vi "Autonomous Independent.vi"() -> ()   [LabVIEW 2015]
doc: "This VI is called when autonomous begins, and will automatically be terminated when autonomous ends. You can carry out timed or sensor driven robot movement independently without needing to return to the caller."
uses:
  <vilib>/Rock Robotics/WPI/Utilities/WPI_GetSetVariantRefNum.vi
  <vilib>/Rock Robotics/Network Tables/NT Write Numeric Array.vi
  <vilib>/Rock Robotics/Network Tables/NT Read String.vi
  Robot Motor Controllers.llb/RobotGlobalVariables.vi
  <vilib>/Rock Robotics/WPI/RobotDrive/WPI_RobotDriveArcadeDrive_Standard(NoSaturation).vi
  <vilib>/Rock Robotics/Network Tables/NT Write Boolean.vi
panel:
  out "Current Movement, for debugging 2":T1 {"Y Joystick Value" scale=1.0..-1.0; "X Joystick Value" scale=-1.0..1.0}
  in  "Array of robot movements 2":T2(array[cluster])=[{"X Joystick Value"=0.39393939393939403, "Y Joystick Value"=0.0, "Delay (sec)"=1.0, "Movement Name"="turn"}, {"X Joystick Value"=-0.3737373737373737, "Y Joystick Value"=0.0, "Delay (sec)"=1.0, "Movement Name"="turn back"}] {"Y Joystick Value" scale=1.0..-1.0; "X Joystick Value" scale=-1.0..1.0}
  out "Current Movement, for debugging":T1 {"Y Joystick Value" scale=1.0..-1.0; "X Joystick Value" scale=-1.0..1.0}
  in  "Array of robot movements":T2(array[cluster])=[{"X Joystick Value"=0.39393939393939403, "Y Joystick Value"=0.0, "Delay (sec)"=1.0, "Movement Name"="turn"}, {"X Joystick Value"=-0.3737373737373737, "Y Joystick Value"=0.0, "Delay (sec)"=1.0, "Movement Name"="turn back"}] {"Y Joystick Value" scale=1.0..-1.0; "X Joystick Value" scale=-1.0..1.0}
  # "Be sure to right-click and choose Data Operations>>Make Current Value default if you want to save the array values with the VI"
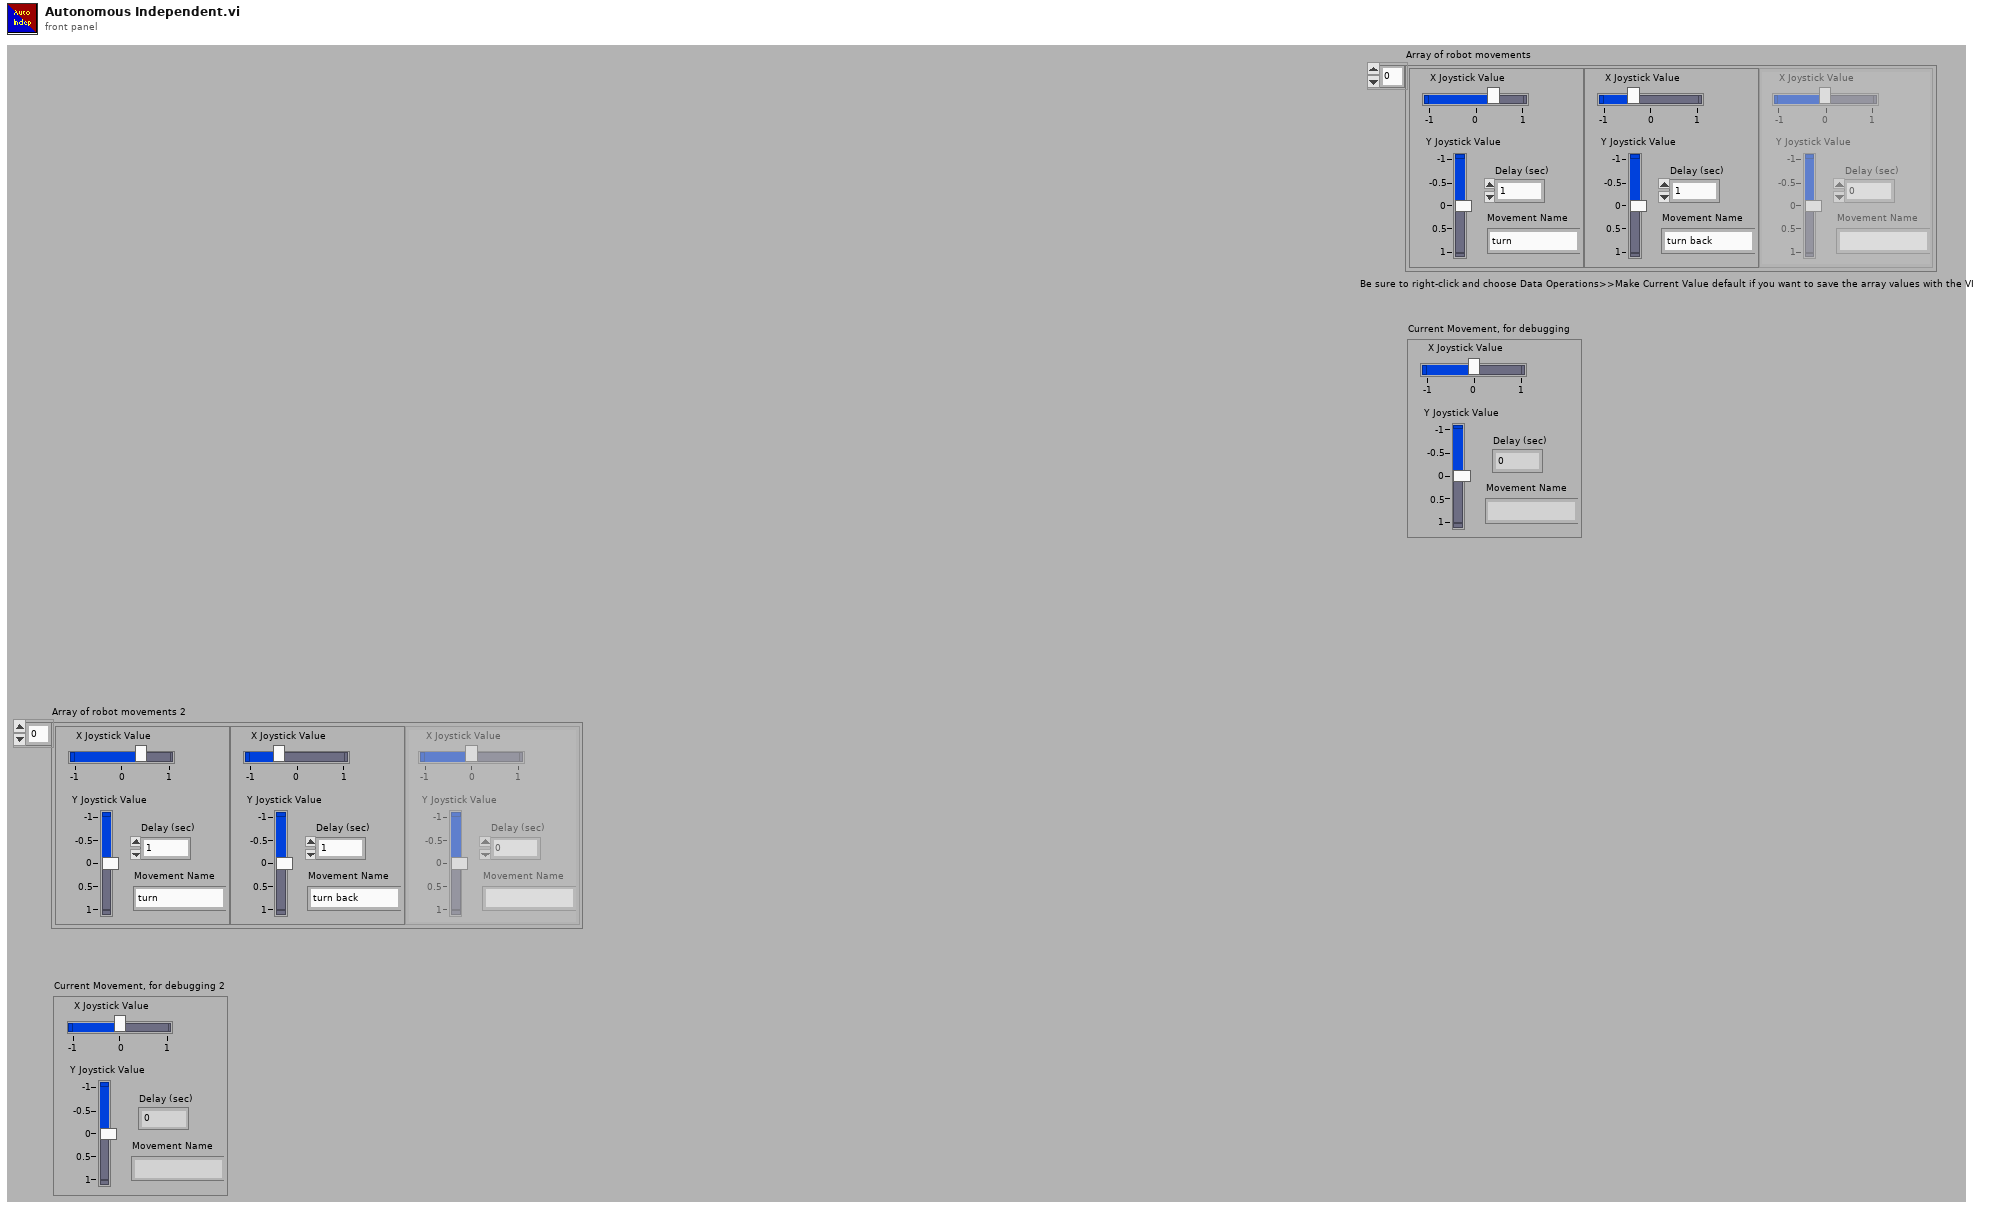
[diagram p1: front panel]
types:
  T1 = cluster{"X Joystick Value":dbl, "Y Joystick Value":dbl, "Delay (sec)":dbl, "Movement Name":string}
  T2 = cluster{"X Joystick Value":dbl, "Y Joystick Value":dbl, "Delay (sec)":dbl, "Movement Name":string}[]
  T3 = typedef "WPI_RobotDriveDevRef.ctl" = cluster{"DevStatus":errorcluster, "Motors[]":T4[], "Square Inputs":bool, "Max Output":dbl}
  T4 = typedef "WPI_MotorControlDeviceRef.ctl" = cluster{"DeviceStatus":errorcluster, "Type":T5, "PWM":cluster{"PWM Channel":T6, "DeadBand":T7}, "CAN":cluster{"Device Number":u8, "Control Mode":T8, "Semaphore":T9, "Max Vout":dbl, "TalonSRX Control Mode":T10}, "Invert":bool}
  T5 = typedef "WPI_MotorControlType.ctl" = enum16{"PWM", "CAN", "CANTalonSRX"}
  T6 = typedef "FPGA_DIOPWMChannel.ctl" = enum8{"PWM 0", "PWM 1", "PWM 2", "PWM 3", "PWM 4", "PWM 5", "PWM 6", "PWM 7", "PWM 8", "PWM 9", "PWM MXP 0", "PWM MXP 1", "PWM MXP 2", "PWM MXP 3", "PWM MXP 4", "PWM MXP 5", "PWM MXP 6", "PWM MXP 7", "PWM MXP 8", "PWM MXP 9", "Invalid"}
  T7 = typedef "WPI_PWMDeadband.ctl" = cluster{"Name":string, "maxPositivePwm":i32, "minPositivePwm":i32, "centerPwm":i32, "maxNegativePwm":i32, "minNegativePwm":i32, "angularRange":u16}
  T8 = typedef "WPI_CANJaguar_ControlMode.ctl" = enum8{"Percent VBus", "Current", "Speed", "Position", "Voltage"}
  T9 = typedef "Semaphore RefNum" = refnum<k1>
  T10 = typedef "WPI_CANTalonSRX_APIControlMode.ctl" = enum8{"Percent VBus", "Speed", "Position", "Slave", "Unchanged / Invalid", "Voltage Compensation", "Current", "Motion Profile"}
  T11 = typedef "WPI_JoystickDevRef.ctl" = cluster{"Device":T12}
  T12 = typedef "WPI_JoystickDeviceEnum.ctl" = enum16{"USB 0", "USB 1", "USB 2", "USB 3", "USB 4", "USB 5"}
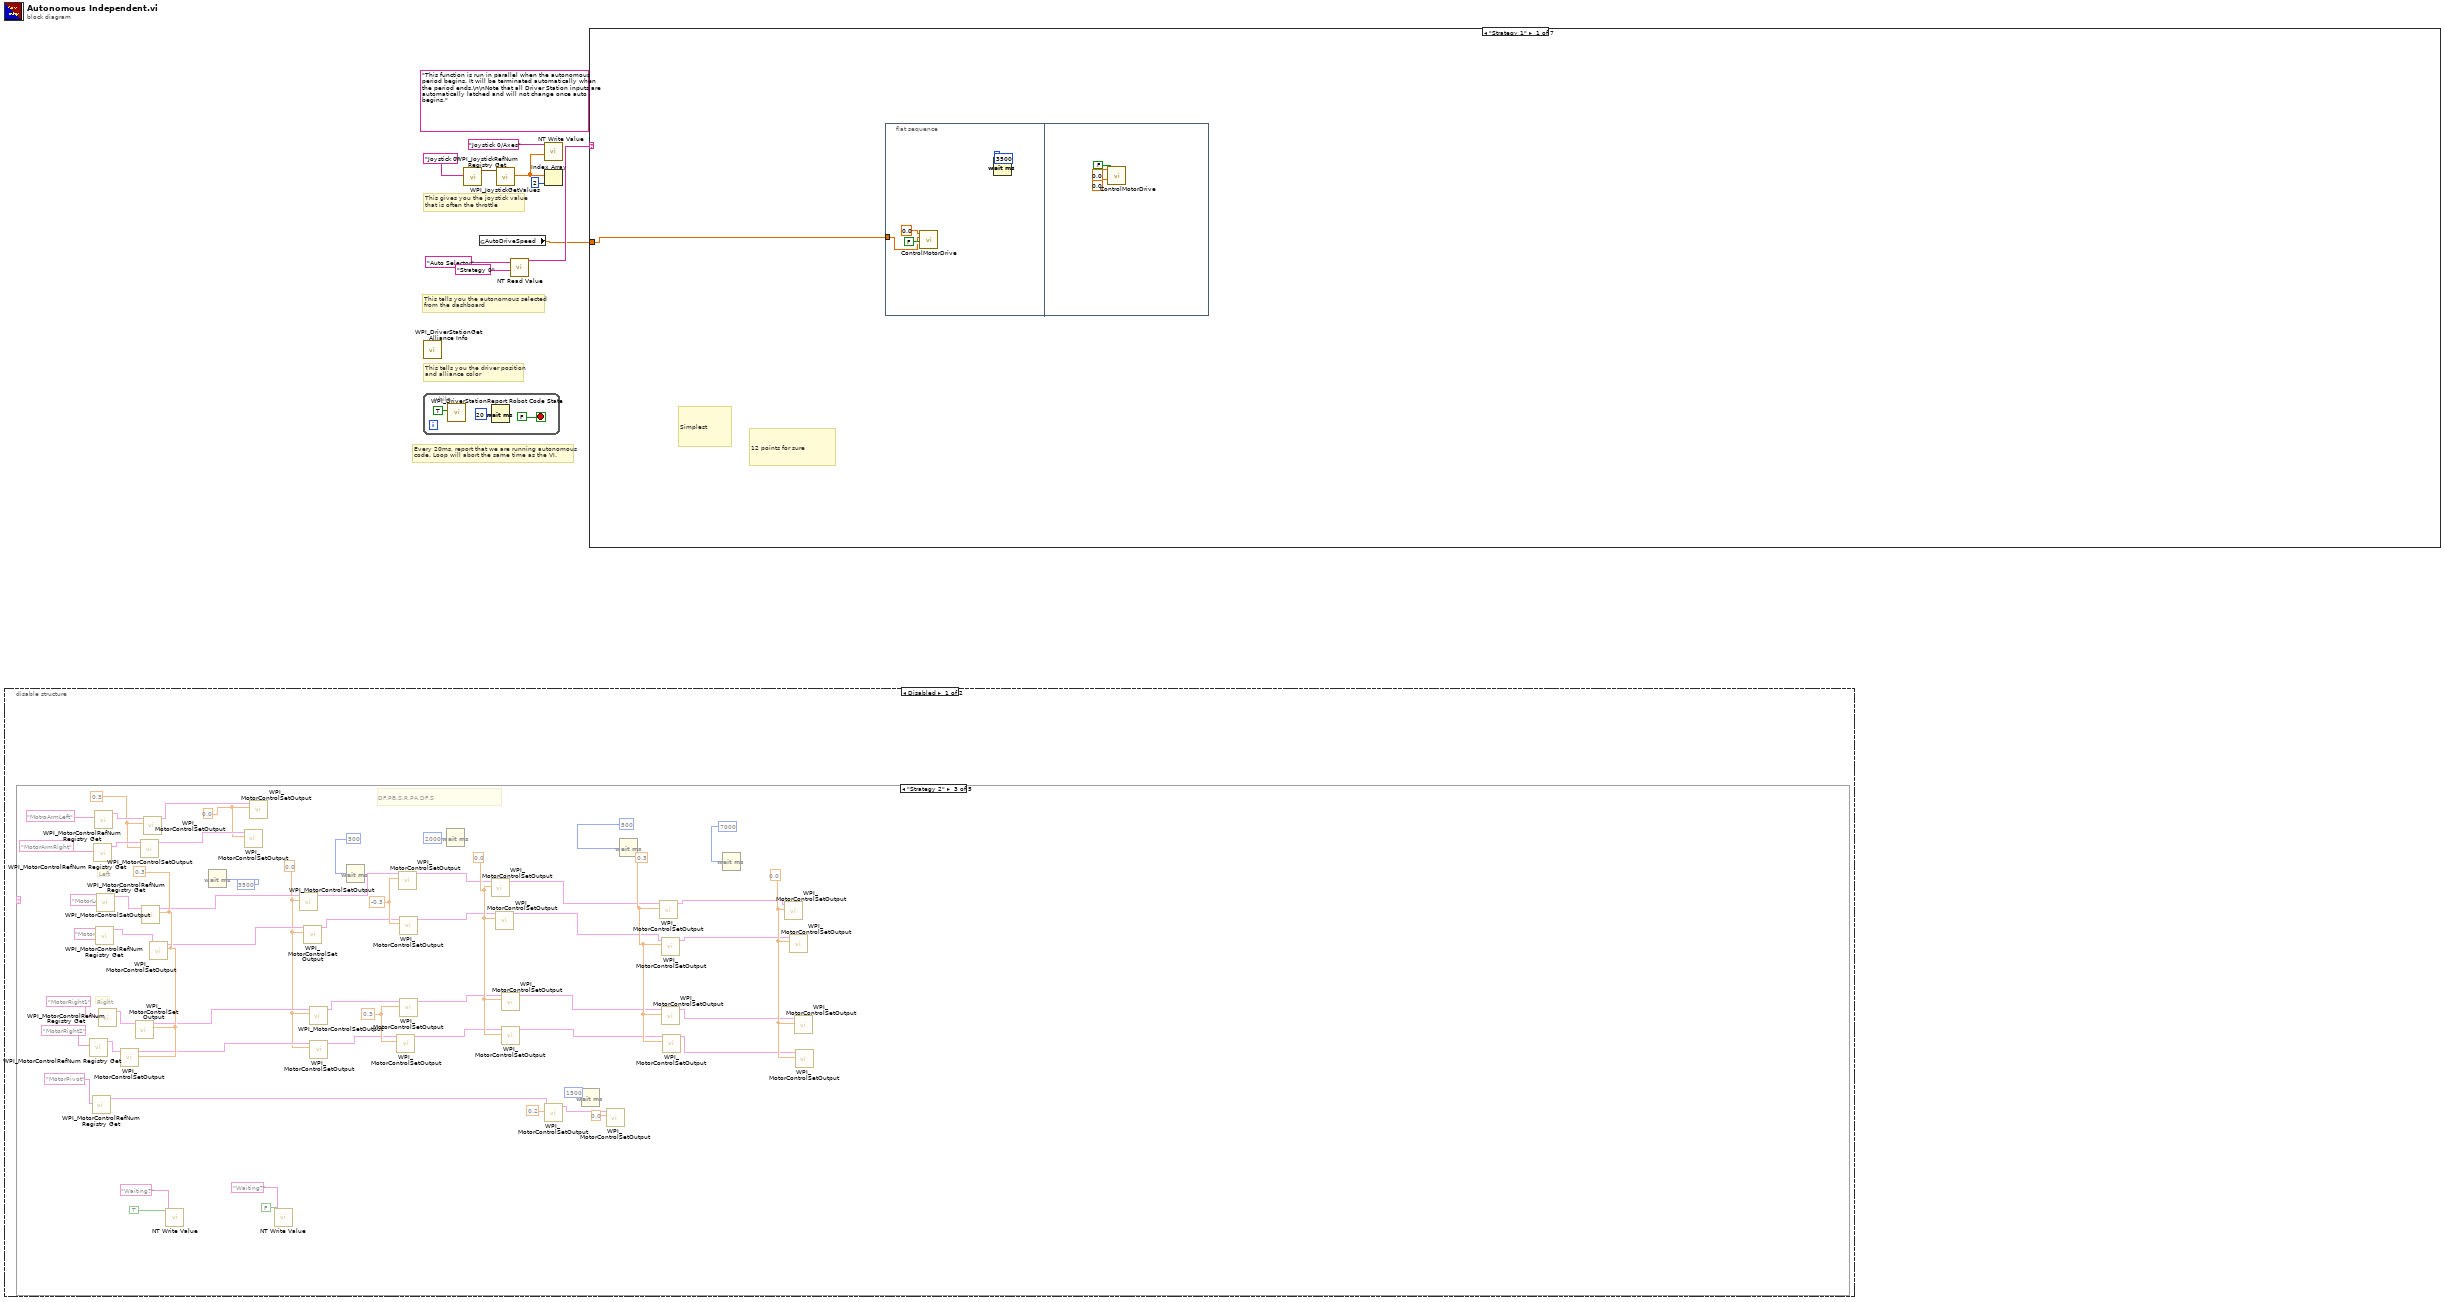
[diagram p0: block diagram]
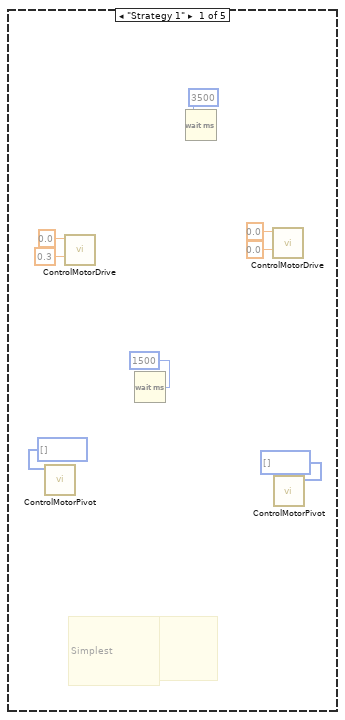
[diagram p2: hidden frame]
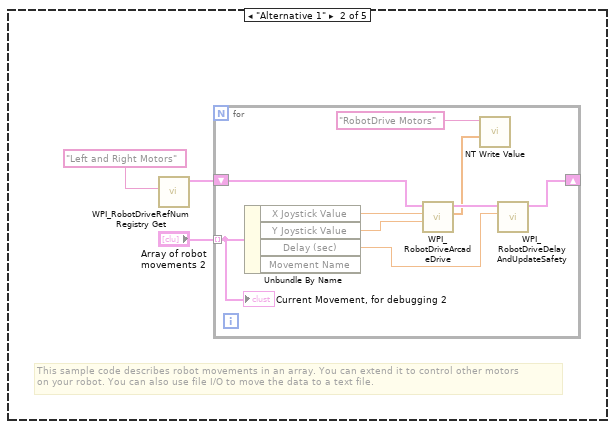
[diagram p3: hidden frame]
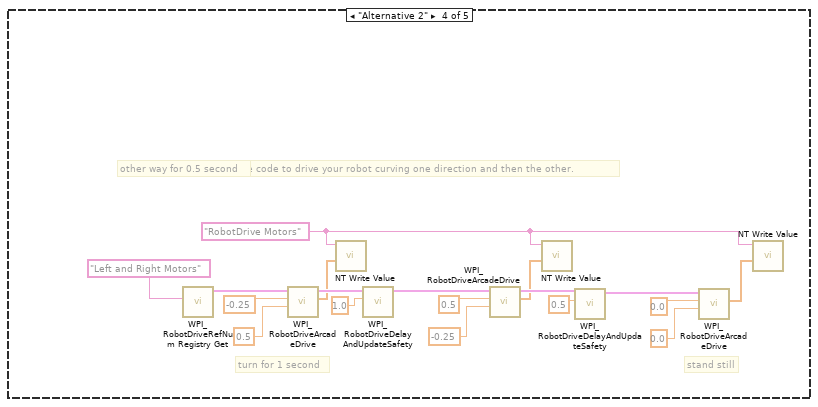
[diagram p4: hidden frame]
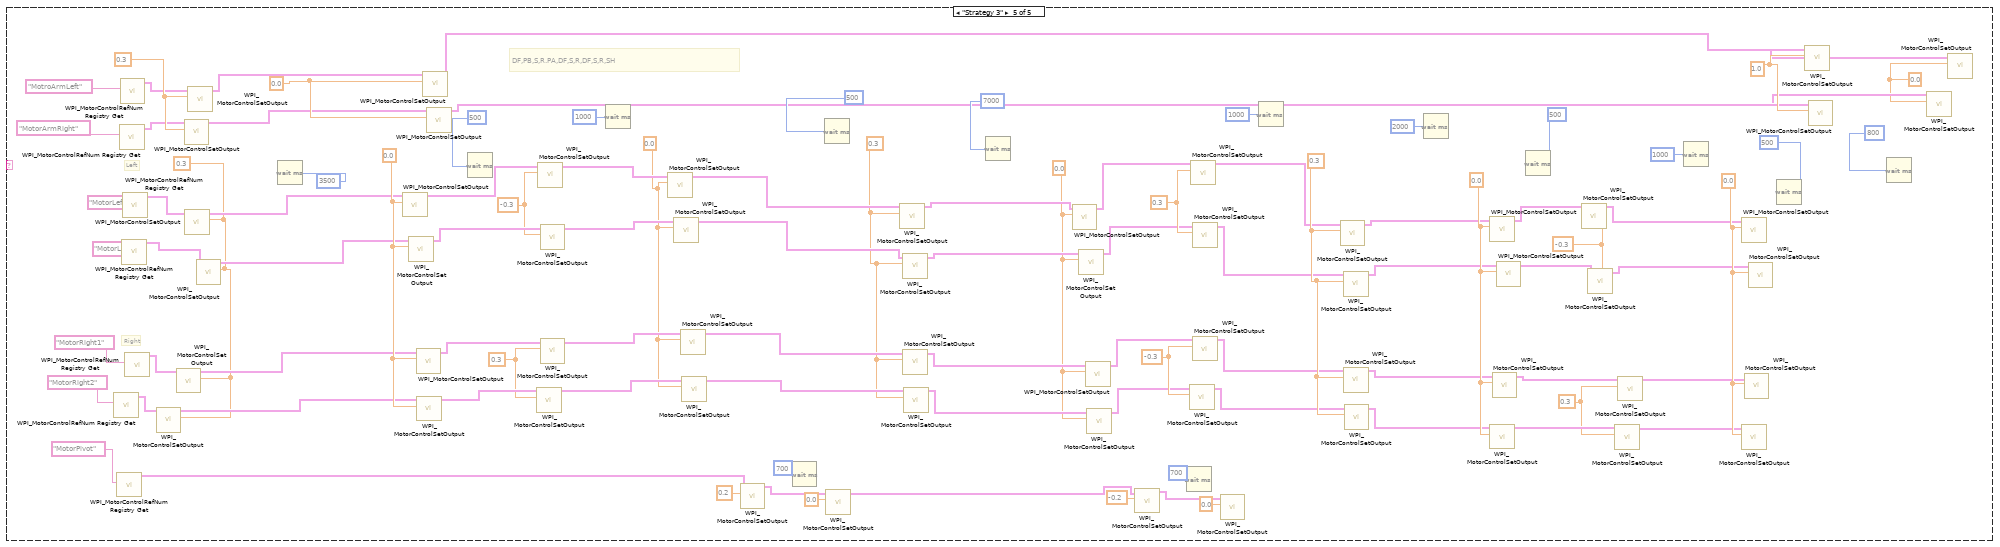
[diagram p5: hidden frame]
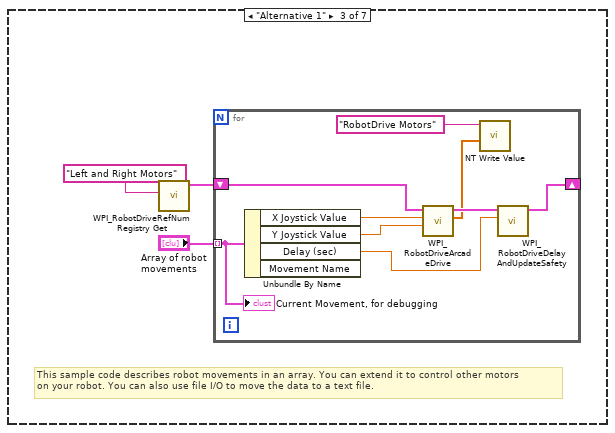
[diagram p8: hidden frame]
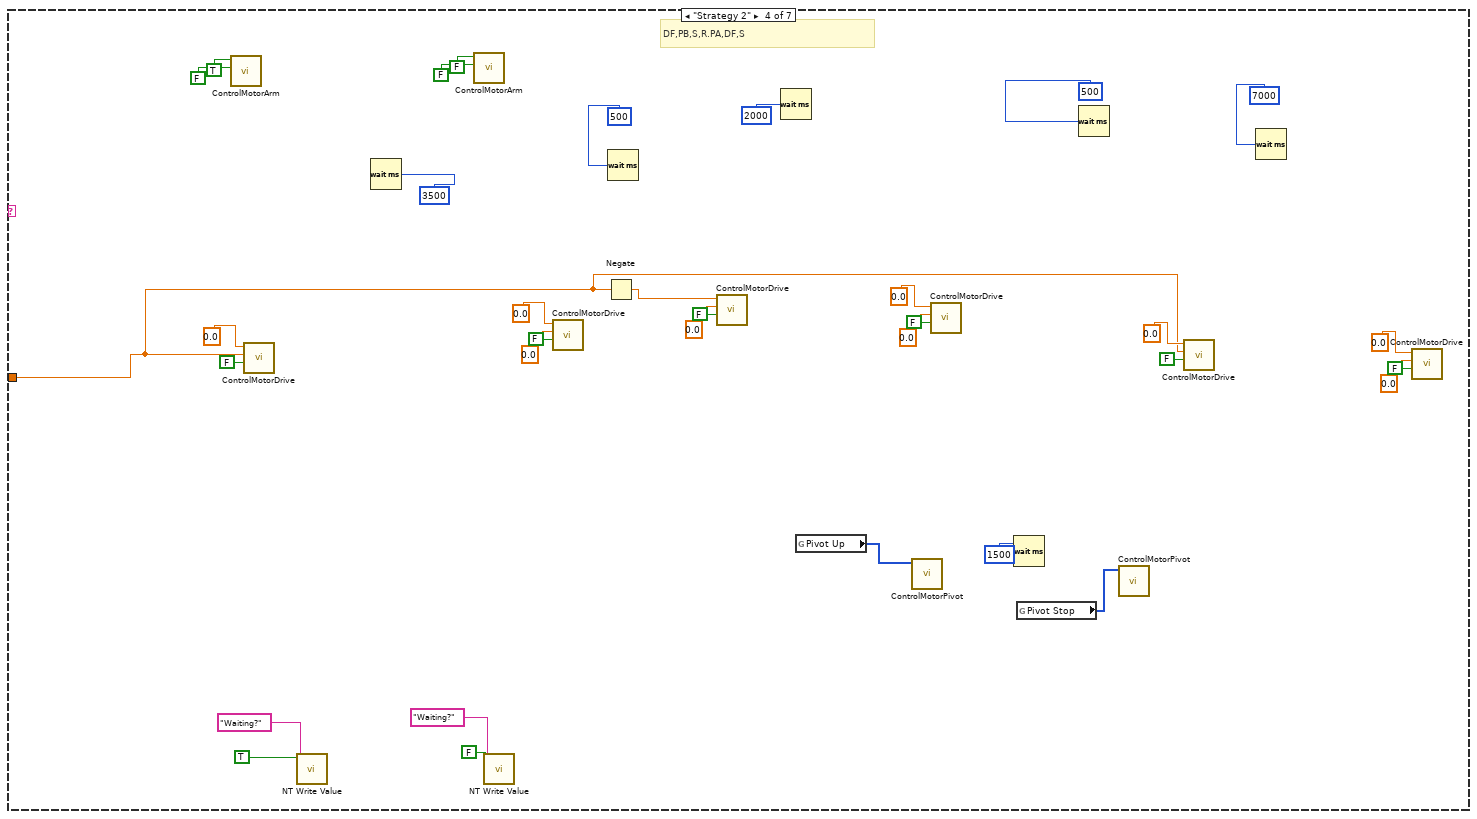
[diagram p9: hidden frame]
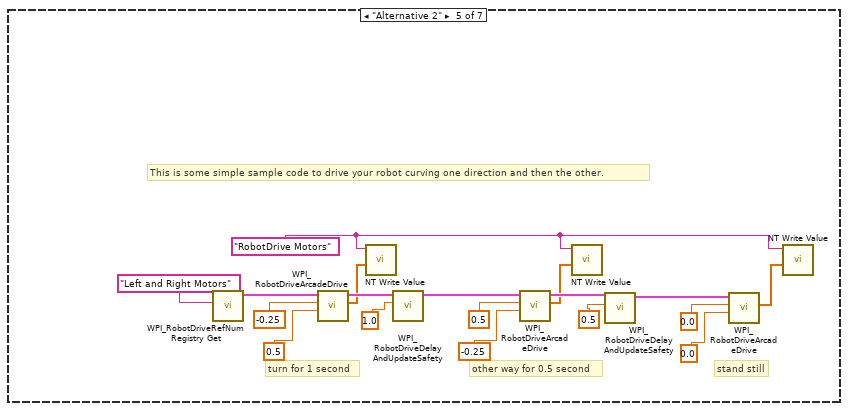
[diagram p10: hidden frame]
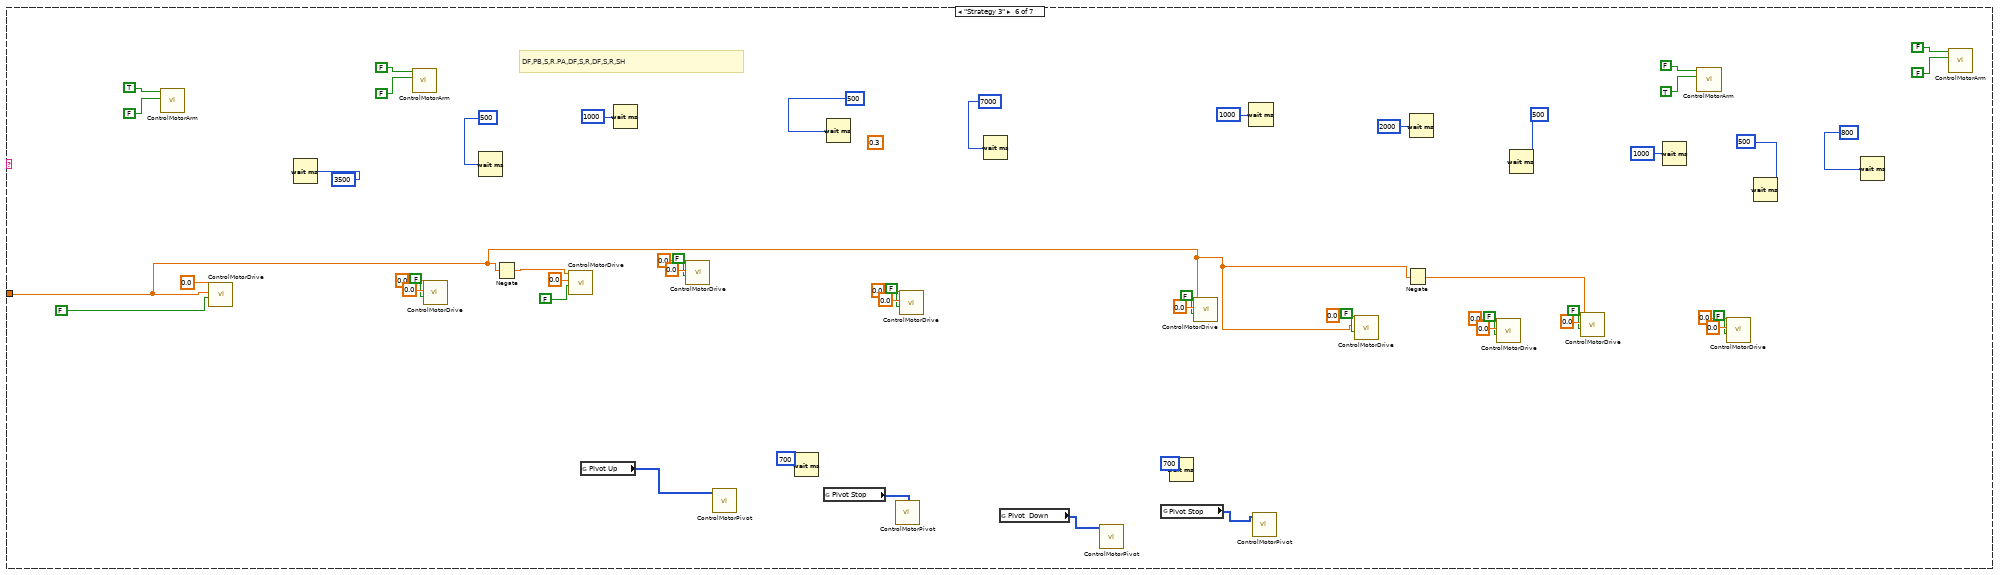
[diagram p11: hidden frame]
diagram:
  (unwired) "This function is run in parallel when the autonomous period begins. It will be terminated automatically when the period ends.\n\nNote that all Driver Station inputs are automatically latched and will not change once auto begins."
  # "This tells you the autonomous selected\nfrom the dashboard"
  # "Every 20ms, report that we are running autonomous\ncode. Loop will abort the same time as the VI."
  # "This gives you the joystick value\nthat is often the throttle"
  # "This tells you the driver position\nand alliance color"
  n1 = disable-structure shown="Disabled" {
    frame Disabled {
      n2 = case shown="\"Strategy 2\"" {
        selector: _ -> [_ _ _ _ _]
        frame "Strategy 1" {
          # "Simplest"
          # "12 points for sure"
          n3 = call "ControlMotorPivot.vi"("POVs"=i16[] []) -> ()  [unwired: 11 in]
          n4 = call "ControlMotorDrive.vi"("Y - Value"=0.3, "X - Value"=0.0) -> ()  [unwired: 10 in]
          n5 = Wait (ms)(milliseconds to wait=u32 1500) -> ()  [unwired: 1 out]
          n6 = Wait (ms)(milliseconds to wait=u32 3500) -> ()  [unwired: 1 out]
          n7 = call "ControlMotorDrive.vi"("Y - Value"=0.0, "X - Value"=0.0) -> ()  [unwired: 10 in]
          n8 = call "ControlMotorPivot.vi"("POVs"=i16[] []) -> ()  [unwired: 11 in]
        }
        frame "Alternative 1" {
          # "This sample code describes robot movements in an array. You can extend it to control other motors\non your robot. You can also use file I/O to move the data to a text file."
          n9 = call <vilib>:"WPI_RobotDriveRefNum Registry Get.vi"("refnum name"="Left and Right Motors") -> ("RobotDriveDevRef"=w19:T3)  [unwired: 1 in, 9 out]
          n10 = for {
            shift-right: [w27] -> _
            shift-left: w19 -> [w28]
            tunnel: "Array of robot movements 2" -> [w23] mode=indexing
            n11 = Unbundle By Name(w23) -> ("X Joystick Value"=w26:dbl, "Y Joystick Value"=w25:dbl, "Delay (sec)"=w24:dbl)  [unwired: 1 out]
            n12 = call-poly <vilib>:"WPI_RobotDriveArcadeDrive.vi"("Y axis value"=w25, "X axis value"=w26, "RobotDriveDevRef"=w28) -> ("Motor Values"=w21:dbl[], "RobotDriveDevRef"=w29:T3)  [unwired: 1 in, 6 out]
            n13 = call-poly <vilib>:"NT Write Value.vi"("Numeric Array"=w21, "Name"="RobotDrive Motors") -> ()  [unwired: 9 in, 1 out]
            n14 = call <vilib>:"WPI_RobotDriveDelayAndUpdateSafety.vi"("Delay (s)"=w24, "RobotDriveDevRef"=w29) -> ("RobotDriveDevRef 2"=w27:T3)  [unwired: 8 in, 1 out]
            "Current Movement, for debugging 2" <- w23
          }
        }
        frame "Strategy 2" {
          w34 = 0.0
          w41 = 0.3 ("Output")
          w46 = 0.0
          w50 = 0.3
          w53 = -0.3
          w59 = 0.0
          w62 = 0.3 ("Output")
          w73 = 0.0
          w83 = 0.3 ("Output")
          # "DF,PB,S,R.PA,DF,S"
          # "Right"
          # "Left"
          n15 = call <vilib>:"WPI_MotorControlRefNum Registry Get.vi"("refnum name"="MotorRight2") -> ("MotorControlDevRef"=w82:T4)  [unwired: 9 in, 1 out]
          n16 = call <vilib>:"WPI_MotorControlRefNum Registry Get.vi"("refnum name"="MotorPivot") -> ("MotorControlDevRef"=w70:T4)  [unwired: 9 in, 1 out]
          n17 = call <vilib>:"WPI_MotorControlRefNum Registry Get.vi"("refnum name"="MotorArmRight") -> ("MotorControlDevRef"=w63:T4)  [unwired: 9 in, 1 out]
          n18 = call <vilib>:"WPI_MotorControlRefNum Registry Get.vi"("refnum name"="MotroArmLeft") -> ("MotorControlDevRef"=w64:T4)  [unwired: 9 in, 1 out]
          n19 = call <vilib>:"WPI_MotorControlRefNum Registry Get.vi"("refnum name"="MotorLeft2") -> ("MotorControlDevRef"=w80:T4)  [unwired: 9 in, 1 out]
          n20 = call <vilib>:"WPI_MotorControlRefNum Registry Get.vi"("refnum name"="MotorLeft1") -> ("MotorControlDevRef"=w79:T4)  [unwired: 9 in, 1 out]
          n21 = call <vilib>:"WPI_MotorControlRefNum Registry Get.vi"("refnum name"="MotorRight1") -> ("MotorControlDevRef"=w81:T4)  [unwired: 9 in, 1 out]
          n22 = call <vilib>:"WPI_MotorControlSetOutput.vi"("Output"=w83, "MotorControlDevRef"=w82) -> ("MotorControlDevRef"=w74:T4)  [unwired: 7 in, 2 out]
          n23 = call <vilib>:"WPI_MotorControlSetOutput.vi"("Output"=w83, "MotorControlDevRef"=w81) -> ("MotorControlDevRef"=w75:T4)  [unwired: 7 in, 2 out]
          n24 = call <vilib>:"WPI_MotorControlSetOutput.vi"("Output"=w62, "MotorControlDevRef"=w63) -> ("MotorControlDevRef"=w60:T4)  [unwired: 7 in, 2 out]
          n25 = call <vilib>:"WPI_MotorControlSetOutput.vi"("Output"=w83, "MotorControlDevRef"=w79) -> ("MotorControlDevRef"=w77:T4)  [unwired: 7 in, 2 out]
          n26 = call <vilib>:"WPI_MotorControlSetOutput.vi"("Output"=w62, "MotorControlDevRef"=w64) -> ("MotorControlDevRef"=w61:T4)  [unwired: 7 in, 2 out]
          n27 = call <vilib>:"WPI_MotorControlSetOutput.vi"("Output"=w83, "MotorControlDevRef"=w80) -> ("MotorControlDevRef"=w76:T4)  [unwired: 7 in, 2 out]
          n28 = call-poly <vilib>:"NT Write Value.vi"("Boolean"=TRUE, "Name"="Waiting?") -> ()  [unwired: 9 in, 1 out]
          n29 = Wait (ms)(milliseconds to wait=u32 3500) -> ()  [unwired: 1 out]
          n30 = call <vilib>:"WPI_MotorControlSetOutput.vi"("Output"=w59, "MotorControlDevRef"=w60) -> ()  [unwired: 7 in, 3 out]
          n31 = call <vilib>:"WPI_MotorControlSetOutput.vi"("Output"=w59, "MotorControlDevRef"=w61) -> ()  [unwired: 7 in, 3 out]
          n32 = call-poly <vilib>:"NT Write Value.vi"("Boolean"=FALSE, "Name"="Waiting?") -> ()  [unwired: 9 in, 1 out]
          n33 = call <vilib>:"WPI_MotorControlSetOutput.vi"("Output"=w73, "MotorControlDevRef"=w77) -> ("MotorControlDevRef"=w51:T4)  [unwired: 7 in, 2 out]
          n34 = call <vilib>:"WPI_MotorControlSetOutput.vi"("Output"=w73, "MotorControlDevRef"=w76) -> ("MotorControlDevRef"=w52:T4)  [unwired: 7 in, 2 out]
          n35 = call <vilib>:"WPI_MotorControlSetOutput.vi"("Output"=w73, "MotorControlDevRef"=w75) -> ("MotorControlDevRef"=w48:T4)  [unwired: 7 in, 2 out]
          n36 = call <vilib>:"WPI_MotorControlSetOutput.vi"("Output"=w73, "MotorControlDevRef"=w74) -> ("MotorControlDevRef"=w49:T4)  [unwired: 7 in, 2 out]
          n37 = Wait (ms)(milliseconds to wait=u32 500) -> ()  [unwired: 1 out]
          n38 = call <vilib>:"WPI_MotorControlSetOutput.vi"("Output"=w50, "MotorControlDevRef"=w49) -> ("MotorControlDevRef"=w42:T4)  [unwired: 7 in, 2 out]
          n39 = call <vilib>:"WPI_MotorControlSetOutput.vi"("Output"=w53, "MotorControlDevRef"=w51) -> ("MotorControlDevRef"=w45:T4)  [unwired: 7 in, 2 out]
          n40 = call <vilib>:"WPI_MotorControlSetOutput.vi"("Output"=w53, "MotorControlDevRef"=w52) -> ("MotorControlDevRef"=w44:T4)  [unwired: 7 in, 2 out]
          n41 = call <vilib>:"WPI_MotorControlSetOutput.vi"("Output"=w50, "MotorControlDevRef"=w48) -> ("MotorControlDevRef"=w43:T4)  [unwired: 7 in, 2 out]
          n42 = Wait (ms)(milliseconds to wait=u32 2000) -> ()  [unwired: 1 out]
          n43 = call <vilib>:"WPI_MotorControlSetOutput.vi"("Output"=w46, "MotorControlDevRef"=w45) -> ("MotorControlDevRef"=w38:T4)  [unwired: 7 in, 2 out]
          n44 = call <vilib>:"WPI_MotorControlSetOutput.vi"("Output"=w46, "MotorControlDevRef"=w44) -> ("MotorControlDevRef"=w37:T4)  [unwired: 7 in, 2 out]
          n45 = call <vilib>:"WPI_MotorControlSetOutput.vi"("Output"=w46, "MotorControlDevRef"=w43) -> ("MotorControlDevRef"=w36:T4)  [unwired: 7 in, 2 out]
          n46 = call <vilib>:"WPI_MotorControlSetOutput.vi"("Output"=w46, "MotorControlDevRef"=w42) -> ("MotorControlDevRef"=w35:T4)  [unwired: 7 in, 2 out]
          n47 = call <vilib>:"WPI_MotorControlSetOutput.vi"("Output"=0.2, "MotorControlDevRef"=w70) -> ("MotorControlDevRef"=w69:T4)  [unwired: 7 in, 2 out]
          n48 = Wait (ms)(milliseconds to wait=u32 1500) -> ()  [unwired: 1 out]
          n49 = call <vilib>:"WPI_MotorControlSetOutput.vi"("Output"=0.0, "MotorControlDevRef"=w69) -> ()  [unwired: 7 in, 3 out]
          n50 = Wait (ms)(milliseconds to wait=u32 500) -> ()  [unwired: 1 out]
          n51 = call <vilib>:"WPI_MotorControlSetOutput.vi"("Output"=w41, "MotorControlDevRef"=w38) -> ("MotorControlDevRef"=w33:T4)  [unwired: 7 in, 2 out]
          n52 = call <vilib>:"WPI_MotorControlSetOutput.vi"("Output"=w41, "MotorControlDevRef"=w37) -> ("MotorControlDevRef"=w32:T4)  [unwired: 7 in, 2 out]
          n53 = call <vilib>:"WPI_MotorControlSetOutput.vi"("Output"=w41, "MotorControlDevRef"=w36) -> ("MotorControlDevRef"=w31:T4)  [unwired: 7 in, 2 out]
          n54 = call <vilib>:"WPI_MotorControlSetOutput.vi"("Output"=w41, "MotorControlDevRef"=w35) -> ("MotorControlDevRef"=w30:T4)  [unwired: 7 in, 2 out]
          n55 = Wait (ms)(milliseconds to wait=u32 7000) -> ()  [unwired: 1 out]
          n56 = call <vilib>:"WPI_MotorControlSetOutput.vi"("Output"=w34, "MotorControlDevRef"=w33) -> ()  [unwired: 7 in, 3 out]
          n57 = call <vilib>:"WPI_MotorControlSetOutput.vi"("Output"=w34, "MotorControlDevRef"=w32) -> ()  [unwired: 7 in, 3 out]
          n58 = call <vilib>:"WPI_MotorControlSetOutput.vi"("Output"=w34, "MotorControlDevRef"=w31) -> ()  [unwired: 7 in, 3 out]
          n59 = call <vilib>:"WPI_MotorControlSetOutput.vi"("Output"=w34, "MotorControlDevRef"=w30) -> ()  [unwired: 7 in, 3 out]
        }
        frame "Alternative 2" {
          w89 = "RobotDrive Motors" ("Name")
          # "This is some simple sample code to drive your robot curving one direction and then the other."
          # "stand still"
          # "other way for 0.5 second"
          # "turn for 1 second"
          n60 = call <vilib>:"WPI_RobotDriveRefNum Registry Get.vi"("refnum name"="Left and Right Motors") -> ("RobotDriveDevRef"=w105:T3)  [unwired: 1 in, 9 out]
          n61 = call-poly <vilib>:"WPI_RobotDriveArcadeDrive.vi"("Y axis value"=0.5 ("X axis value"), "X axis value"=-0.25, "RobotDriveDevRef"=w105) -> ("Motor Values"=w88:dbl[], "RobotDriveDevRef"=w98:T3)  [unwired: 1 in, 6 out]
          n62 = call-poly <vilib>:"NT Write Value.vi"("Numeric Array"=w88, "Name"=w89) -> ()  [unwired: 9 in, 1 out]
          n63 = call <vilib>:"WPI_RobotDriveDelayAndUpdateSafety.vi"("Delay (s)"=1.0, "RobotDriveDevRef"=w98) -> ("RobotDriveDevRef 2"=w99:T3)  [unwired: 8 in, 1 out]
          n64 = call-poly <vilib>:"WPI_RobotDriveArcadeDrive.vi"("Y axis value"=-0.25 ("X axis value"), "X axis value"=0.5, "RobotDriveDevRef"=w99) -> ("Motor Values"=w90:dbl[], "RobotDriveDevRef"=w100:T3)  [unwired: 1 in, 6 out]
          n65 = call-poly <vilib>:"NT Write Value.vi"("Numeric Array"=w90, "Name"=w89) -> ()  [unwired: 9 in, 1 out]
          n66 = call <vilib>:"WPI_RobotDriveDelayAndUpdateSafety.vi"("Delay (s)"=0.5, "RobotDriveDevRef"=w100) -> ("RobotDriveDevRef 2"=w101:T3)  [unwired: 8 in, 1 out]
          n67 = call-poly <vilib>:"WPI_RobotDriveArcadeDrive.vi"("Y axis value"=0.0 ("X axis value"), "X axis value"=0.0, "RobotDriveDevRef"=w101) -> ("Motor Values"=w91:dbl[])  [unwired: 1 in, 7 out]
          n68 = call-poly <vilib>:"NT Write Value.vi"("Numeric Array"=w91, "Name"=w89) -> ()  [unwired: 9 in, 1 out]
        }
        frame "Strategy 3" {
          w113 = 0.0
          w106 = 0.0
          w119 = 1.0
          w108 = 0.3
          w124 = -0.3
          w131 = 0.0
          w137 = 0.3 ("Output")
          w143 = -0.3
          w142 = 0.3
          w199 = 0.0
          w192 = 0.3 ("Output")
          w187 = 0.0
          w183 = 0.3
          w180 = -0.3
          w178 = 0.0
          w175 = 0.3 ("Output")
          w164 = 0.0
          w154 = 0.3 ("Output")
          # "DF,PB,S,R.PA,DF,S,R,DF,S,R,SH"
          # "Right"
          # "Left"
          n69 = call <vilib>:"WPI_MotorControlRefNum Registry Get.vi"("refnum name"="MotorRight2") -> ("MotorControlDevRef"=w155:T4)  [unwired: 9 in, 1 out]
          n70 = call <vilib>:"WPI_MotorControlRefNum Registry Get.vi"("refnum name"="MotorPivot") -> ("MotorControlDevRef"=w167:T4)  [unwired: 9 in, 1 out]
          n71 = call <vilib>:"WPI_MotorControlRefNum Registry Get.vi"("refnum name"="MotorArmRight") -> ("MotorControlDevRef"=w174:T4)  [unwired: 9 in, 1 out]
          n72 = call <vilib>:"WPI_MotorControlRefNum Registry Get.vi"("refnum name"="MotroArmLeft") -> ("MotorControlDevRef"=w173:T4)  [unwired: 9 in, 1 out]
          n73 = call <vilib>:"WPI_MotorControlRefNum Registry Get.vi"("refnum name"="MotorLeft2") -> ("MotorControlDevRef"=w157:T4)  [unwired: 9 in, 1 out]
          n74 = call <vilib>:"WPI_MotorControlRefNum Registry Get.vi"("refnum name"="MotorLeft1") -> ("MotorControlDevRef"=w158:T4)  [unwired: 9 in, 1 out]
          n75 = call <vilib>:"WPI_MotorControlRefNum Registry Get.vi"("refnum name"="MotorRight1") -> ("MotorControlDevRef"=w156:T4)  [unwired: 9 in, 1 out]
          n76 = call <vilib>:"WPI_MotorControlSetOutput.vi"("Output"=w154, "MotorControlDevRef"=w155) -> ("MotorControlDevRef"=w163:T4)  [unwired: 7 in, 2 out]
          n77 = call <vilib>:"WPI_MotorControlSetOutput.vi"("Output"=w154, "MotorControlDevRef"=w156) -> ("MotorControlDevRef"=w162:T4)  [unwired: 7 in, 2 out]
          n78 = call <vilib>:"WPI_MotorControlSetOutput.vi"("Output"=w175, "MotorControlDevRef"=w174) -> ("MotorControlDevRef"=w177:T4)  [unwired: 7 in, 2 out]
          n79 = call <vilib>:"WPI_MotorControlSetOutput.vi"("Output"=w154, "MotorControlDevRef"=w158) -> ("MotorControlDevRef"=w160:T4)  [unwired: 7 in, 2 out]
          n80 = call <vilib>:"WPI_MotorControlSetOutput.vi"("Output"=w175, "MotorControlDevRef"=w173) -> ("MotorControlDevRef"=w176:T4)  [unwired: 7 in, 2 out]
          n81 = call <vilib>:"WPI_MotorControlSetOutput.vi"("Output"=w154, "MotorControlDevRef"=w157) -> ("MotorControlDevRef"=w161:T4)  [unwired: 7 in, 2 out]
          n82 = Wait (ms)(milliseconds to wait=u32 3500) -> ()  [unwired: 1 out]
          n83 = call <vilib>:"WPI_MotorControlSetOutput.vi"("Output"=w164, "MotorControlDevRef"=w160) -> ("MotorControlDevRef"=w182:T4)  [unwired: 7 in, 2 out]
          n84 = call <vilib>:"WPI_MotorControlSetOutput.vi"("Output"=w164, "MotorControlDevRef"=w161) -> ("MotorControlDevRef"=w181:T4)  [unwired: 7 in, 2 out]
          n85 = call <vilib>:"WPI_MotorControlSetOutput.vi"("Output"=w164, "MotorControlDevRef"=w162) -> ("MotorControlDevRef"=w185:T4)  [unwired: 7 in, 2 out]
          n86 = call <vilib>:"WPI_MotorControlSetOutput.vi"("Output"=w164, "MotorControlDevRef"=w163) -> ("MotorControlDevRef"=w184:T4)  [unwired: 7 in, 2 out]
          n87 = call <vilib>:"WPI_MotorControlSetOutput.vi"("Output"=w178, "MotorControlDevRef"=w176) -> ("MotorControlDevRef"=w118:T4)  [unwired: 7 in, 2 out]
          n88 = call <vilib>:"WPI_MotorControlSetOutput.vi"("Output"=w178, "MotorControlDevRef"=w177) -> ("MotorControlDevRef"=w117:T4)  [unwired: 7 in, 2 out]
          n89 = Wait (ms)(milliseconds to wait=u32 500) -> ()  [unwired: 1 out]
          n90 = call <vilib>:"WPI_MotorControlSetOutput.vi"("Output"=w183, "MotorControlDevRef"=w184) -> ("MotorControlDevRef"=w191:T4)  [unwired: 7 in, 2 out]
          n91 = call <vilib>:"WPI_MotorControlSetOutput.vi"("Output"=w180, "MotorControlDevRef"=w182) -> ("MotorControlDevRef"=w188:T4)  [unwired: 7 in, 2 out]
          n92 = call <vilib>:"WPI_MotorControlSetOutput.vi"("Output"=w180, "MotorControlDevRef"=w181) -> ("MotorControlDevRef"=w189:T4)  [unwired: 7 in, 2 out]
          n93 = call <vilib>:"WPI_MotorControlSetOutput.vi"("Output"=w183, "MotorControlDevRef"=w185) -> ("MotorControlDevRef"=w190:T4)  [unwired: 7 in, 2 out]
          n94 = Wait (ms)(milliseconds to wait=u32 1000) -> ()  [unwired: 1 out]
          n95 = call <vilib>:"WPI_MotorControlSetOutput.vi"("Output"=w187, "MotorControlDevRef"=w188) -> ("MotorControlDevRef"=w195:T4)  [unwired: 7 in, 2 out]
          n96 = call <vilib>:"WPI_MotorControlSetOutput.vi"("Output"=w187, "MotorControlDevRef"=w189) -> ("MotorControlDevRef"=w196:T4)  [unwired: 7 in, 2 out]
          n97 = call <vilib>:"WPI_MotorControlSetOutput.vi"("Output"=w187, "MotorControlDevRef"=w190) -> ("MotorControlDevRef"=w197:T4)  [unwired: 7 in, 2 out]
          n98 = call <vilib>:"WPI_MotorControlSetOutput.vi"("Output"=w187, "MotorControlDevRef"=w191) -> ("MotorControlDevRef"=w198:T4)  [unwired: 7 in, 2 out]
          n99 = call <vilib>:"WPI_MotorControlSetOutput.vi"("Output"=0.2, "MotorControlDevRef"=w167) -> ("MotorControlDevRef"=w168:T4)  [unwired: 7 in, 2 out]
          n100 = Wait (ms)(milliseconds to wait=u32 700) -> ()  [unwired: 1 out]
          n101 = Wait (ms)(milliseconds to wait=u32 500) -> ()  [unwired: 1 out]
          n102 = call <vilib>:"WPI_MotorControlSetOutput.vi"("Output"=0.0, "MotorControlDevRef"=w168) -> ("MotorControlDevRef"=w145:T4)  [unwired: 7 in, 2 out]
          n103 = call <vilib>:"WPI_MotorControlSetOutput.vi"("Output"=w192, "MotorControlDevRef"=w195) -> ("MotorControlDevRef"=w200:T4)  [unwired: 7 in, 2 out]
          n104 = call <vilib>:"WPI_MotorControlSetOutput.vi"("Output"=w192, "MotorControlDevRef"=w196) -> ("MotorControlDevRef"=w201:T4)  [unwired: 7 in, 2 out]
          n105 = call <vilib>:"WPI_MotorControlSetOutput.vi"("Output"=w192, "MotorControlDevRef"=w197) -> ("MotorControlDevRef"=w202:T4)  [unwired: 7 in, 2 out]
          n106 = call <vilib>:"WPI_MotorControlSetOutput.vi"("Output"=w192, "MotorControlDevRef"=w198) -> ("MotorControlDevRef"=w203:T4)  [unwired: 7 in, 2 out]
          n107 = Wait (ms)(milliseconds to wait=u32 7000) -> ()  [unwired: 1 out]
          n108 = call <vilib>:"WPI_MotorControlSetOutput.vi"("Output"=w199, "MotorControlDevRef"=w200) -> ("MotorControlDevRef"=w141:T4)  [unwired: 7 in, 2 out]
          n109 = call <vilib>:"WPI_MotorControlSetOutput.vi"("Output"=w199, "MotorControlDevRef"=w201) -> ("MotorControlDevRef"=w140:T4)  [unwired: 7 in, 2 out]
          n110 = call <vilib>:"WPI_MotorControlSetOutput.vi"("Output"=w199, "MotorControlDevRef"=w202) -> ("MotorControlDevRef"=w139:T4)  [unwired: 7 in, 2 out]
          n111 = call <vilib>:"WPI_MotorControlSetOutput.vi"("Output"=w199, "MotorControlDevRef"=w203) -> ("MotorControlDevRef"=w138:T4)  [unwired: 7 in, 2 out]
          n112 = call <vilib>:"WPI_MotorControlSetOutput.vi"("Output"=-0.2, "MotorControlDevRef"=w145) -> ("MotorControlDevRef"=w147:T4)  [unwired: 7 in, 2 out]
          n113 = Wait (ms)(milliseconds to wait=u32 700) -> ()  [unwired: 1 out]
          n114 = call <vilib>:"WPI_MotorControlSetOutput.vi"("Output"=w143, "MotorControlDevRef"=w138) -> ("MotorControlDevRef"=w133:T4)  [unwired: 7 in, 2 out]
          n115 = call <vilib>:"WPI_MotorControlSetOutput.vi"("Output"=w142, "MotorControlDevRef"=w141) -> ("MotorControlDevRef"=w136:T4)  [unwired: 7 in, 2 out]
          n116 = call <vilib>:"WPI_MotorControlSetOutput.vi"("Output"=w142, "MotorControlDevRef"=w140) -> ("MotorControlDevRef"=w135:T4)  [unwired: 7 in, 2 out]
          n117 = call <vilib>:"WPI_MotorControlSetOutput.vi"("Output"=w143, "MotorControlDevRef"=w139) -> ("MotorControlDevRef"=w134:T4)  [unwired: 7 in, 2 out]
          n118 = call <vilib>:"WPI_MotorControlSetOutput.vi"("Output"=0.0, "MotorControlDevRef"=w147) -> ()  [unwired: 7 in, 3 out]
          n119 = Wait (ms)(milliseconds to wait=u32 1000) -> ()  [unwired: 1 out]
          n120 = call <vilib>:"WPI_MotorControlSetOutput.vi"("Output"=w137, "MotorControlDevRef"=w136) -> ("MotorControlDevRef"=w130:T4)  [unwired: 7 in, 2 out]
          n121 = call <vilib>:"WPI_MotorControlSetOutput.vi"("Output"=w137, "MotorControlDevRef"=w135) -> ("MotorControlDevRef"=w129:T4)  [unwired: 7 in, 2 out]
          n122 = call <vilib>:"WPI_MotorControlSetOutput.vi"("Output"=w137, "MotorControlDevRef"=w134) -> ("MotorControlDevRef"=w128:T4)  [unwired: 7 in, 2 out]
          n123 = call <vilib>:"WPI_MotorControlSetOutput.vi"("Output"=w137, "MotorControlDevRef"=w133) -> ("MotorControlDevRef"=w127:T4)  [unwired: 7 in, 2 out]
          n124 = Wait (ms)(milliseconds to wait=u32 2000) -> ()  [unwired: 1 out]
          n125 = call <vilib>:"WPI_MotorControlSetOutput.vi"("Output"=w131, "MotorControlDevRef"=w130) -> ("MotorControlDevRef"=w123:T4)  [unwired: 7 in, 2 out]
          n126 = call <vilib>:"WPI_MotorControlSetOutput.vi"("Output"=w131, "MotorControlDevRef"=w127) -> ("MotorControlDevRef"=w120:T4)  [unwired: 7 in, 2 out]
          n127 = call <vilib>:"WPI_MotorControlSetOutput.vi"("Output"=w131, "MotorControlDevRef"=w128) -> ("MotorControlDevRef"=w121:T4)  [unwired: 7 in, 2 out]
          n128 = call <vilib>:"WPI_MotorControlSetOutput.vi"("Output"=w131, "MotorControlDevRef"=w129) -> ("MotorControlDevRef"=w122:T4)  [unwired: 7 in, 2 out]
          n129 = Wait (ms)(milliseconds to wait=u32 500) -> ()  [unwired: 1 out]
          n130 = call <vilib>:"WPI_MotorControlSetOutput.vi"("Output"=w124, "MotorControlDevRef"=w123) -> ("MotorControlDevRef"=w112:T4)  [unwired: 7 in, 2 out]
          n131 = call <vilib>:"WPI_MotorControlSetOutput.vi"("Output"=w124, "MotorControlDevRef"=w122) -> ("MotorControlDevRef"=w111:T4)  [unwired: 7 in, 2 out]
          n132 = call <vilib>:"WPI_MotorControlSetOutput.vi"("Output"=w108, "MotorControlDevRef"=w120) -> ("MotorControlDevRef"=w109:T4)  [unwired: 7 in, 2 out]
          n133 = call <vilib>:"WPI_MotorControlSetOutput.vi"("Output"=w108, "MotorControlDevRef"=w121) -> ("MotorControlDevRef"=w110:T4)  [unwired: 7 in, 2 out]
          n134 = Wait (ms)(milliseconds to wait=u32 1000) -> ()  [unwired: 1 out]
          n135 = call <vilib>:"WPI_MotorControlSetOutput.vi"("Output"=w113, "MotorControlDevRef"=w112) -> ()  [unwired: 7 in, 3 out]
          n136 = call <vilib>:"WPI_MotorControlSetOutput.vi"("Output"=w113, "MotorControlDevRef"=w109) -> ()  [unwired: 7 in, 3 out]
          n137 = call <vilib>:"WPI_MotorControlSetOutput.vi"("Output"=w113, "MotorControlDevRef"=w110) -> ()  [unwired: 7 in, 3 out]
          n138 = call <vilib>:"WPI_MotorControlSetOutput.vi"("Output"=w113, "MotorControlDevRef"=w111) -> ()  [unwired: 7 in, 3 out]
          n139 = Wait (ms)(milliseconds to wait=u32 500) -> ()  [unwired: 1 out]
          n140 = call <vilib>:"WPI_MotorControlSetOutput.vi"("Output"=w119, "MotorControlDevRef"=w118) -> ("MotorControlDevRef"=w115:T4)  [unwired: 7 in, 2 out]
          n141 = call <vilib>:"WPI_MotorControlSetOutput.vi"("Output"=w119, "MotorControlDevRef"=w117) -> ("MotorControlDevRef"=w114:T4)  [unwired: 7 in, 2 out]
          n142 = Wait (ms)(milliseconds to wait=u32 800) -> ()  [unwired: 1 out]
          n143 = call <vilib>:"WPI_MotorControlSetOutput.vi"("Output"=w106, "MotorControlDevRef"=w114) -> ()  [unwired: 7 in, 3 out]
          n144 = call <vilib>:"WPI_MotorControlSetOutput.vi"("Output"=w106, "MotorControlDevRef"=w115) -> ()  [unwired: 7 in, 3 out]
        }
      }
    }
    frame Enabled {
    }
  }
  n145 = while {
    stop <- FALSE stop-if-true
    n146 = call <vilib>:"WPI_DriverStationReport Robot Code State.vi"("Autonomous"=TRUE) -> ()  [unwired: 10 in, 1 out]
    n147 = Wait (ms)(milliseconds to wait=u32 20) -> ()  [unwired: 1 out]
  }
  n148 = call <vilib>:"WPI_DriverStationGet Alliance Info.vi"() -> ()  [unwired: 12 out]
  n149 = call <vilib>:"WPI_JoystickRefNum Registry Get.vi"("refnum name"="Joystick 0") -> ("JoystickDevRef"=w8:T11)  [unwired: 1 in, 9 out]
  n150 = global read "RobotGlobalVariables.vi" "AutoDriveSpeed"() -> (w2:dbl)
  n151 = call <vilib>:"WPI_JoystickGetValues.vi"("JoystickDevRef"=w8) -> ("Axes"=w4:dbl[])  [unwired: 6 in, 4 out]
  n152 = call-poly <vilib>:"NT Read Value.vi"("Default Value"="Strategy 0", "Name"="Auto Selector") -> ("String"=w5:string)  [unwired: 8 in, 1 out]
  n153 = call-poly <vilib>:"NT Write Value.vi"("Numeric Array"=w4, "Name"="Joystick 0/Axes") -> ()  [unwired: 9 in, 1 out]
  n154 = Index Array(array=w4, index=2) -> ()  [unwired: 1 out]
  n155 = case shown="\"Strategy 1\"" w5 {
    tunnel: w2 -> [w207 _ _ w227 _ w278 _]
    frame "Strategy 1" {
      # "Simplest"
      # "12 points for sure"
      n156 = flat-sequence {
        tunnel: w207 -> [w209]
        frame #0 {
          n157 = call "ControlMotorDrive.vi"("Use Deadzone"=FALSE, "Y - Value"=w209, "X - Value"=0.0) -> ()  [unwired: 9 in]
          n158 = Wait (ms)(milliseconds to wait=u32 3500) -> ()  [unwired: 1 out]
        }
        frame #1 {
          n159 = call "ControlMotorDrive.vi"("Use Deadzone"=FALSE, "Y - Value"=0.0, "X - Value"=0.0) -> ()  [unwired: 9 in]
        }
      }
    }
    frame "Strategy 0", Default {
    }
    frame "Alternative 1" {
      # "This sample code describes robot movements in an array. You can extend it to control other motors\non your robot. You can also use file I/O to move the data to a text file."
      n160 = call <vilib>:"WPI_RobotDriveRefNum Registry Get.vi"("refnum name"="Left and Right Motors") -> ("RobotDriveDevRef"=w216:T3)  [unwired: 1 in, 9 out]
      n161 = for {
        shift-right: [w224] -> _
        shift-left: w216 -> [w225]
        tunnel: "Array of robot movements" -> [w220] mode=indexing
        n162 = Unbundle By Name(w220) -> ("X Joystick Value"=w223:dbl, "Y Joystick Value"=w222:dbl, "Delay (sec)"=w221:dbl)  [unwired: 1 out]
        n163 = call-poly <vilib>:"WPI_RobotDriveArcadeDrive.vi"("Y axis value"=w222, "X axis value"=w223, "RobotDriveDevRef"=w225) -> ("Motor Values"=w218:dbl[], "RobotDriveDevRef"=w226:T3)  [unwired: 1 in, 6 out]
        n164 = call-poly <vilib>:"NT Write Value.vi"("Numeric Array"=w218, "Name"="RobotDrive Motors") -> ()  [unwired: 9 in, 1 out]
        n165 = call <vilib>:"WPI_RobotDriveDelayAndUpdateSafety.vi"("Delay (s)"=w221, "RobotDriveDevRef"=w226) -> ("RobotDriveDevRef 2"=w224:T3)  [unwired: 8 in, 1 out]
        "Current Movement, for debugging" <- w220
      }
    }
    frame "Strategy 2" {
      # "DF,PB,S,R.PA,DF,S"
      n166 = call "ControlMotorArm.vi"("Shooting"=FALSE, "Feeding"=TRUE) -> ()  [unwired: 10 in]
      n167 = call "ControlMotorDrive.vi"("Use Deadzone"=FALSE, "Y - Value"=w227, "X - Value"=0.0) -> ()  [unwired: 9 in]
      n168 = call-poly <vilib>:"NT Write Value.vi"("Boolean"=TRUE, "Name"="Waiting?") -> ()  [unwired: 9 in, 1 out]
      n169 = Wait (ms)(milliseconds to wait=u32 3500) -> ()  [unwired: 1 out]
      n170 = call "ControlMotorArm.vi"("Shooting"=FALSE, "Feeding"=FALSE) -> ()  [unwired: 10 in]
      n171 = call-poly <vilib>:"NT Write Value.vi"("Boolean"=FALSE, "Name"="Waiting?") -> ()  [unwired: 9 in, 1 out]
      n172 = call "ControlMotorDrive.vi"("Use Deadzone"=FALSE, "Y - Value"=0.0, "X - Value"=0.0) -> ()  [unwired: 9 in]
      n173 = Negate(x=w227) -> (-x=w228:dbl)
      n174 = Wait (ms)(milliseconds to wait=u32 500) -> ()  [unwired: 1 out]
      n175 = call "ControlMotorDrive.vi"("Use Deadzone"=FALSE, "Y - Value"=0.0, "X - Value"=w228) -> ()  [unwired: 9 in]
      n176 = Wait (ms)(milliseconds to wait=u32 2000) -> ()  [unwired: 1 out]
      n177 = global read "RobotGlobalVariables.vi" "Pivot Up"() -> (w236:i32[])
      n178 = call "ControlMotorPivot.vi"("POVs"=w236) -> ()  [unwired: 11 in]
      n179 = call "ControlMotorDrive.vi"("Use Deadzone"=FALSE, "Y - Value"=0.0, "X - Value"=0.0) -> ()  [unwired: 9 in]
      n180 = Wait (ms)(milliseconds to wait=u32 1500) -> ()  [unwired: 1 out]
      n181 = global read "RobotGlobalVariables.vi" "Pivot Stop"() -> (w235:i32[])
      n182 = Wait (ms)(milliseconds to wait=u32 500) -> ()  [unwired: 1 out]
      n183 = call "ControlMotorPivot.vi"("POVs"=w235) -> ()  [unwired: 11 in]
      n184 = call "ControlMotorDrive.vi"("Use Deadzone"=FALSE, "Y - Value"=w227, "X - Value"=0.0) -> ()  [unwired: 9 in]
      n185 = Wait (ms)(milliseconds to wait=u32 7000) -> ()  [unwired: 1 out]
      n186 = call "ControlMotorDrive.vi"("Use Deadzone"=FALSE, "Y - Value"=0.0, "X - Value"=0.0) -> ()  [unwired: 9 in]
    }
    frame "Alternative 2" {
      w261 = "RobotDrive Motors" ("Name")
      # "This is some simple sample code to drive your robot curving one direction and then the other."
      # "stand still"
      # "other way for 0.5 second"
      # "turn for 1 second"
      n187 = call <vilib>:"WPI_RobotDriveRefNum Registry Get.vi"("refnum name"="Left and Right Motors") -> ("RobotDriveDevRef"=w277:T3)  [unwired: 1 in, 9 out]
      n188 = call-poly <vilib>:"WPI_RobotDriveArcadeDrive.vi"("Y axis value"=0.5 ("X axis value"), "X axis value"=-0.25, "RobotDriveDevRef"=w277) -> ("Motor Values"=w260:dbl[], "RobotDriveDevRef"=w270:T3)  [unwired: 1 in, 6 out]
      n189 = call-poly <vilib>:"NT Write Value.vi"("Numeric Array"=w260, "Name"=w261) -> ()  [unwired: 9 in, 1 out]
      n190 = call <vilib>:"WPI_RobotDriveDelayAndUpdateSafety.vi"("Delay (s)"=1.0, "RobotDriveDevRef"=w270) -> ("RobotDriveDevRef 2"=w271:T3)  [unwired: 8 in, 1 out]
      n191 = call-poly <vilib>:"WPI_RobotDriveArcadeDrive.vi"("Y axis value"=-0.25 ("X axis value"), "X axis value"=0.5, "RobotDriveDevRef"=w271) -> ("Motor Values"=w262:dbl[], "RobotDriveDevRef"=w272:T3)  [unwired: 1 in, 6 out]
      n192 = call-poly <vilib>:"NT Write Value.vi"("Numeric Array"=w262, "Name"=w261) -> ()  [unwired: 9 in, 1 out]
      n193 = call <vilib>:"WPI_RobotDriveDelayAndUpdateSafety.vi"("Delay (s)"=0.5, "RobotDriveDevRef"=w272) -> ("RobotDriveDevRef 2"=w273:T3)  [unwired: 8 in, 1 out]
      n194 = call-poly <vilib>:"WPI_RobotDriveArcadeDrive.vi"("Y axis value"=0.0 ("X axis value"), "X axis value"=0.0, "RobotDriveDevRef"=w273) -> ("Motor Values"=w263:dbl[])  [unwired: 1 in, 7 out]
      n195 = call-poly <vilib>:"NT Write Value.vi"("Numeric Array"=w263, "Name"=w261) -> ()  [unwired: 9 in, 1 out]
    }
    frame "Strategy 3" {
      (unwired) 0.3 ("Output")
      # "DF,PB,S,R.PA,DF,S,R,DF,S,R,SH"
      n196 = call "ControlMotorArm.vi"("Shooting"=FALSE, "Feeding"=TRUE) -> ()  [unwired: 10 in]
      n197 = call "ControlMotorDrive.vi"("Use Deadzone"=FALSE, "Y - Value"=w278, "X - Value"=0.0) -> ()  [unwired: 9 in]
      n198 = Wait (ms)(milliseconds to wait=u32 3500) -> ()  [unwired: 1 out]
      n199 = call "ControlMotorArm.vi"("Shooting"=FALSE, "Feeding"=FALSE) -> ()  [unwired: 10 in]
      n200 = call "ControlMotorDrive.vi"("Use Deadzone"=FALSE, "Y - Value"=0.0, "X - Value"=0.0) -> ()  [unwired: 9 in]
      n201 = Wait (ms)(milliseconds to wait=u32 500) -> ()  [unwired: 1 out]
      n202 = Negate(x=w278) -> (-x=w280:dbl)
      n203 = call "ControlMotorDrive.vi"("Use Deadzone"=FALSE, "Y - Value"=0.0, "X - Value"=w280) -> ()  [unwired: 9 in]
      n204 = global read "RobotGlobalVariables.vi" "Pivot Up"() -> (w293:i32[])
      n205 = Wait (ms)(milliseconds to wait=u32 1000) -> ()  [unwired: 1 out]
      n206 = call "ControlMotorDrive.vi"("Use Deadzone"=FALSE, "Y - Value"=0.0, "X - Value"=0.0) -> ()  [unwired: 9 in]
      n207 = call "ControlMotorPivot.vi"("POVs"=w293) -> ()  [unwired: 11 in]
      n208 = Wait (ms)(milliseconds to wait=u32 700) -> ()  [unwired: 1 out]
      n209 = global read "RobotGlobalVariables.vi" "Pivot Stop"() -> (w292:i32[])
      n210 = Wait (ms)(milliseconds to wait=u32 500) -> ()  [unwired: 1 out]
      n211 = call "ControlMotorPivot.vi"("POVs"=w292) -> ()  [unwired: 11 in]
      n212 = call "ControlMotorDrive.vi"("Use Deadzone"=FALSE, "Y - Value"=0.0, "X - Value"=0.0) -> ()  [unwired: 9 in]
      n213 = Wait (ms)(milliseconds to wait=u32 7000) -> ()  [unwired: 1 out]
      n214 = global read "RobotGlobalVariables.vi" "Pivot  Down"() -> (w291:i32[])
      n215 = call "ControlMotorPivot.vi"("POVs"=w291) -> ()  [unwired: 11 in]
      n216 = global read "RobotGlobalVariables.vi" "Pivot Stop"() -> (w290:i32[])
      n217 = Wait (ms)(milliseconds to wait=u32 700) -> ()  [unwired: 1 out]
      n218 = call "ControlMotorDrive.vi"("Use Deadzone"=FALSE, "Y - Value"=0.0, "X - Value"=w278) -> ()  [unwired: 9 in]
      n219 = Wait (ms)(milliseconds to wait=u32 1000) -> ()  [unwired: 1 out]
      n220 = call "ControlMotorPivot.vi"("POVs"=w290) -> ()  [unwired: 11 in]
      n221 = call "ControlMotorDrive.vi"("Use Deadzone"=FALSE, "Y - Value"=w278, "X - Value"=0.0) -> ()  [unwired: 9 in]
      n222 = Negate(x=w278) -> (-x=w279:dbl)
      n223 = Wait (ms)(milliseconds to wait=u32 2000) -> ()  [unwired: 1 out]
      n224 = call "ControlMotorDrive.vi"("Use Deadzone"=FALSE, "Y - Value"=0.0, "X - Value"=0.0) -> ()  [unwired: 9 in]
      n225 = Wait (ms)(milliseconds to wait=u32 500) -> ()  [unwired: 1 out]
      n226 = call "ControlMotorDrive.vi"("Use Deadzone"=FALSE, "Y - Value"=0.0, "X - Value"=w279) -> ()  [unwired: 9 in]
      n227 = Wait (ms)(milliseconds to wait=u32 1000) -> ()  [unwired: 1 out]
      n228 = call "ControlMotorArm.vi"("Shooting"=TRUE, "Feeding"=FALSE) -> ()  [unwired: 10 in]
      n229 = call "ControlMotorDrive.vi"("Use Deadzone"=FALSE, "Y - Value"=0.0, "X - Value"=0.0) -> ()  [unwired: 9 in]
      n230 = Wait (ms)(milliseconds to wait=u32 500) -> ()  [unwired: 1 out]
      n231 = Wait (ms)(milliseconds to wait=u32 800) -> ()  [unwired: 1 out]
      n232 = call "ControlMotorArm.vi"("Shooting"=FALSE, "Feeding"=FALSE) -> ()  [unwired: 10 in]
    }
    frame "Strategy 4" {
    }
  }
